vi "2_2.vi"() -> ()   [LabVIEW 2017]
panel:
  out "Bound":dbl
  out "Inverse":dbl
  out "Random*100-50":dbl
  out "Random Number (0~10)":dbl
  out "Negation":dbl
  out "Square":dbl
  out "abs(x)":dbl
  out "Sqrt(x)":dbl
  out "Round to Nearest Function":dbl
  out "Root(x)":dbl
  out "Round Towards +Infinity":dbl
  out "Round Towards -Infinity":dbl
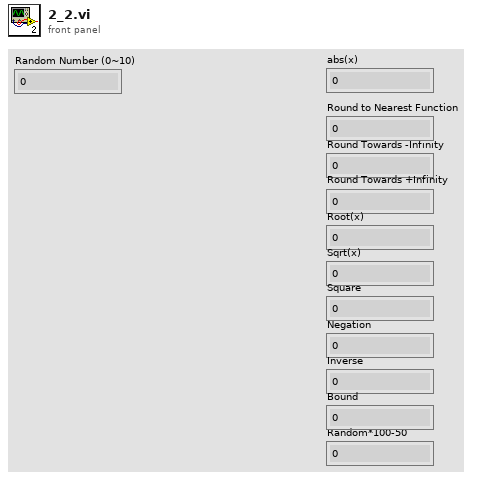
[diagram p1: front panel]
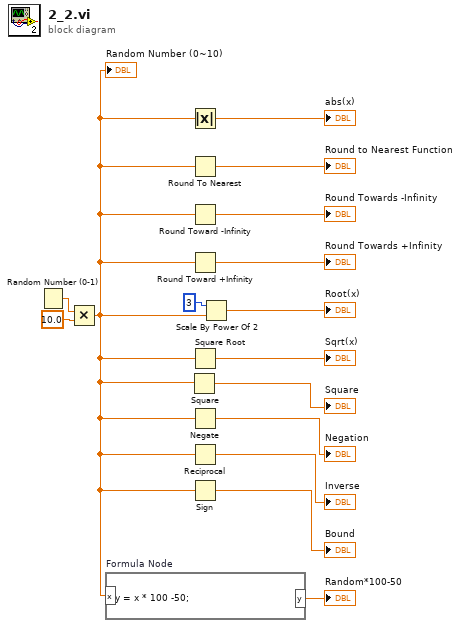
[diagram p0: block diagram]
diagram:
  n1 = Random Number (0-1)() -> (number: 0 to 1=w15:dbl)
  n2 = Multiply(x=w15, y=10.0) -> (x*y=w2:dbl)
  "Random Number (0~10)" <- w2
  n3 = formula code="y = x * 100 -50;"("x"=w2) -> ("y"=→"Random*100-50":dbl)
  n4 = Square(x=w2) -> (x^2=→"Square":dbl)
  n5 = Absolute Value(x=w2) -> (abs(x)=→"abs(x)":dbl)
  n6 = Round To Nearest(number=w2) -> (nearest integer value=→"Round to Nearest Function":dbl)
  n7 = Round Toward -Infinity(1:w2) -> (0:→"Round Towards -Infinity":dbl)
  n8 = Round Toward +Infinity(x=w2) -> (ceil(x): smallest int >= x=→"Round Towards +Infinity":dbl)
  n9 = Square Root(x=w2) -> (sqrt(x)=→"Sqrt(x)":dbl)
  n10 = Negate(x=w2) -> (-x=→"Negation":dbl)
  n11 = Reciprocal(x=w2) -> (1/x=→"Inverse":dbl)
  n12 = Sign(1:w2) -> (0:→"Bound":dbl)
  n13 = Scale By Power Of 2(n=i16 3, x=w2) -> (x*2^n=→"Root(x)":dbl)
